vi "CALIBRATE.vi"(8 "error in (no error)":errorcluster, 9 "string_pot_slope_IN":dbl=1.5 format="%.2f", 10 "pressure_slope_IN":dbl=23.33 format="%.2f", 11 "flow_slope_IN":dbl=51.35 format="%.2f") -> (0 "error out":errorcluster, 1 "string_pot_slope_OUT":dbl=1.5 format="%.2f", 2 "pressure_slope_OUT":dbl=23.33 format="%.2f", 3 "flow_slope_OUT":dbl=51.35 format="%.2f")   [LabVIEW 2016]
panel:
  in  "exit":bool
  in  "string_pot":bool
  in  "pressure":bool
  in  "flow":bool
  in  "start path":path=path "C:/"
  in  "all":bool
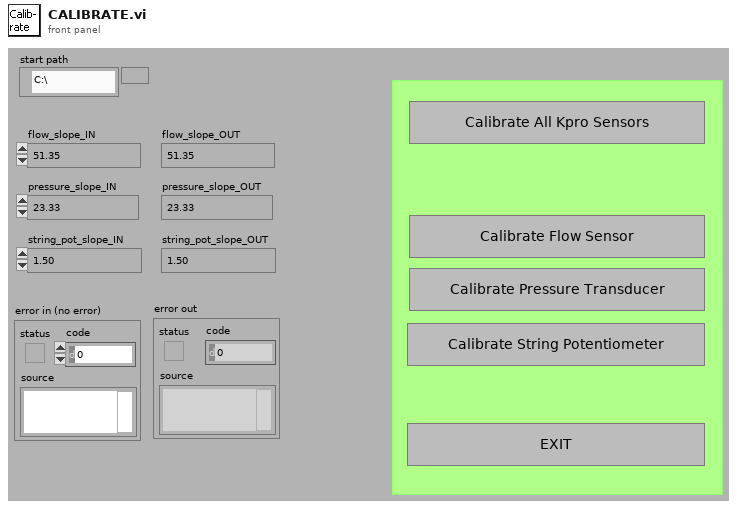
[diagram p1: front panel]
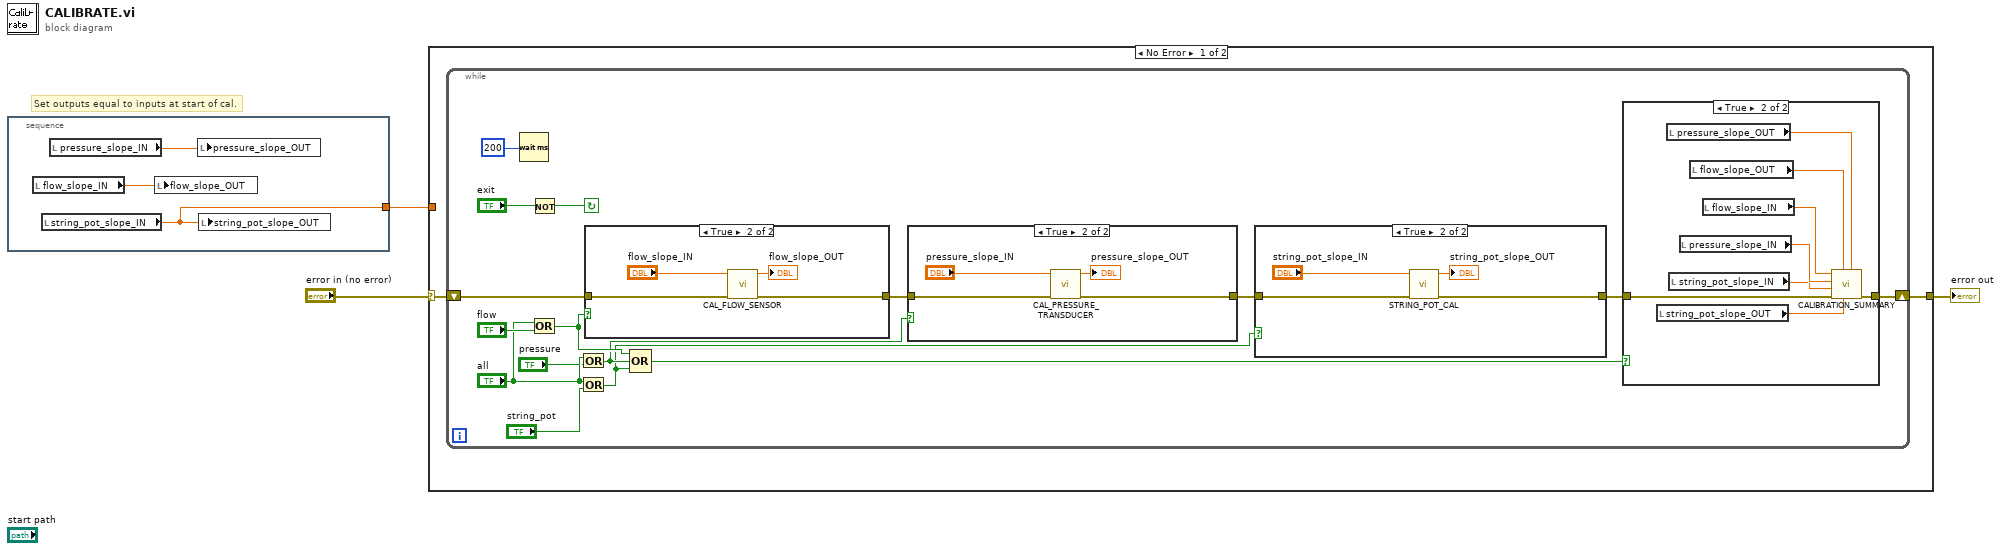
[diagram p0: block diagram]
diagram:
  # "Set outputs equal to inputs at start of cal."
  n1 = stacked-sequence {
    tunnel: [w4] -> w1
    frame #0 {
      n2 = local read "flow_slope_IN"() -> (w6:dbl)
      n3 = local read "string_pot_slope_IN"() -> (w4:dbl)
      n4 = local read "pressure_slope_IN"() -> (w5:dbl)
      n5 = local write "flow_slope_OUT"(w6) -> ()
      n6 = local write "pressure_slope_OUT"(w5) -> ()
      n7 = local write "string_pot_slope_OUT"(w4) -> ()
    }
  }
  n8 = case shown="No Error" "error in (no error)" {
    selector: "error in (no error)" -> [w8 w49]
    tunnel: [w7 w49] -> w2
    tunnel: w1 -> [_ _]
    frame No Error {
      n9 = while {
        shift-left: w8 -> [w21]
        shift-right: [w13] -> w7
        stop <- w24 continue-if-true
        n10 = Wait (ms)(milliseconds to wait=u32 200) -> ()  [unwired: 1 out]
        n11 = Not(x="exit") -> (.not. x?=w24:bool)
        n12 = Or(x="all", y="flow") -> (x .or. y?=w12:bool)
        n13 = Or(x="all", y="pressure") -> (x .or. y?=w11:bool)
        n14 = Or(x="all", y="string_pot") -> (x .or. y?=w10:bool)
        n15 = case shown="True" w12 {
          tunnel: w21 -> [w44 w48]
          tunnel: [w44 w47] -> w18
          frame False {
          }
          frame True {
            n16 = call "CAL_FLOW_SENSOR.vi"("error in (no error)"=w48, "flow_slope_IN"="flow_slope_IN") -> ("error out"=w47:errorcluster, "flow_slope_OUT"=→"flow_slope_OUT":dbl)  [unwired: 8 in]
          }
        }
        n17 = Compound Arithmetic op=OR(w12, w11, w10) -> (w9:bool)
        n18 = case shown="True" w11 {
          tunnel: [w39 w42] -> w19
          tunnel: w18 -> [w39 w43]
          frame False {
          }
          frame True {
            n19 = call "CAL_PRESSURE_TRANSDUCER.vi"("error in (no error)"=w43, "pressure_slope_IN"="pressure_slope_IN") -> ("error out"=w42:errorcluster, "pressure_slope_OUT"=→"pressure_slope_OUT":dbl)  [unwired: 8 in]
          }
        }
        n20 = case shown="True" w10 {
          tunnel: w19 -> [w34 w37]
          tunnel: [w34 w36] -> w14
          frame False {
          }
          frame True {
            n21 = call "STRING_POT_CAL.vi"("error in (no error)"=w37, "string_pot_slope_IN"="string_pot_slope_IN") -> ("error out"=w36:errorcluster, "string_pot_slope_OUT"=→"string_pot_slope_OUT":dbl)  [unwired: 8 in]
          }
        }
        n22 = case shown="True" w9 {
          tunnel: w14 -> [w25 w33]
          tunnel: [w25 w32] -> w13
          frame False {
          }
          frame True {
            n23 = local read "string_pot_slope_OUT"() -> (w26:dbl)
            n24 = local read "pressure_slope_OUT"() -> (w31:dbl)
            n25 = local read "string_pot_slope_IN"() -> (w27:dbl)
            n26 = local read "pressure_slope_IN"() -> (w28:dbl)
            n27 = local read "flow_slope_OUT"() -> (w30:dbl)
            n28 = local read "flow_slope_IN"() -> (w29:dbl)
            n29 = call "CALIBRATION_SUMMARY.vi"("pressure_slope_OUT"=w31, "string_pot_slope_OUT"=w26, "flow_slope_OUT"=w30, "error in (no error)"=w33, "string_pot_slope_IN"=w27, "pressure_slope_IN"=w28, "flow_slope_IN"=w29) -> ("error out"=w32:errorcluster)  [unwired: 4 in]
          }
        }
      }
    }
    frame Error {
    }
  }
  "error out" <- w2
